vi "Write Mode.vi"(8 "error in (no error)":errorcluster, 10 "Mode":enum16{"Pulse", "Sine"}(ring), 11 "RFSoC Driver in":refnum<class "RFSoC Driver.lvclass">) -> (0 "error out":errorcluster, 3 "RFSoC Driver out":refnum<class "RFSoC Driver.lvclass">)   [LabVIEW 2019, in "RFSoC Driver.lvclass"]
uses:
  RFSoC Driver.lvclass
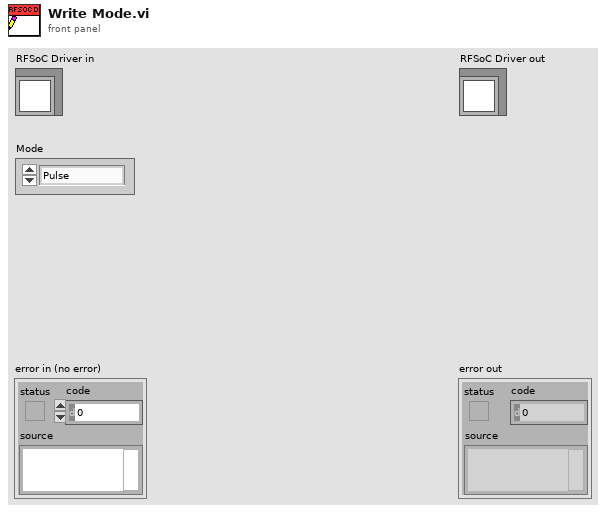
[diagram p1: front panel]
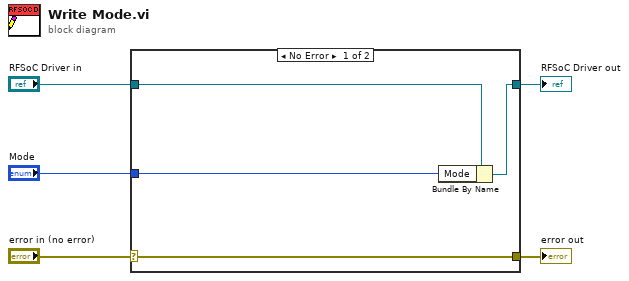
[diagram p0: block diagram]
diagram:
  n1 = case shown="No Error" "error in (no error)" {
    selector: "error in (no error)" -> [w9 w10]
    tunnel: [w9 w10] -> w4
    tunnel: [w7 w11] -> w2
    tunnel: "RFSoC Driver in" -> [w8 w11]
    tunnel: "Mode" -> [w6 _]
    frame No Error {
      n2 = Bundle By Name(cluster=w8, "Mode"=w6) -> (w7:refnum<class "RFSoC Driver.lvclass">)
    }
    frame Error {
    }
  }
  "error out" <- w4
  "RFSoC Driver out" <- w2
